vi "Set Config.vi"(8 "error in (no error)":errorcluster, 9 "Variant":variant, 11 "SJ-210 in":refnum<class "SJ-210.lvclass">) -> (0 "error out":errorcluster, 3 "SJ-210 out":refnum<class "SJ-210.lvclass">)   [LabVIEW 2014, in "SJ-210.lvlib" / "SJ-210.lvclass"]
uses:
  SJ-210.lvclass
  SJ-210.lvclass/SJ-210.ctl
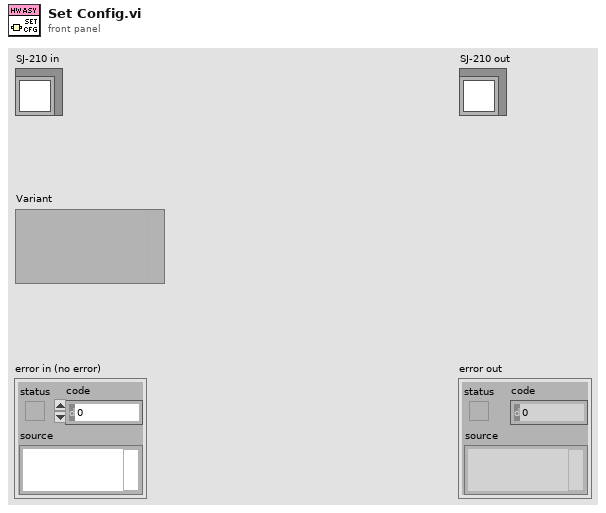
[diagram p1: front panel]
types:
  T1 = cluster{"VISA resource name":refnum<visa-resource-name>}
  T2 = cluster{"Conection Data":cluster{"VISA resource name":refnum<visa-resource-name>}, "ACQ Data":dbl[]}
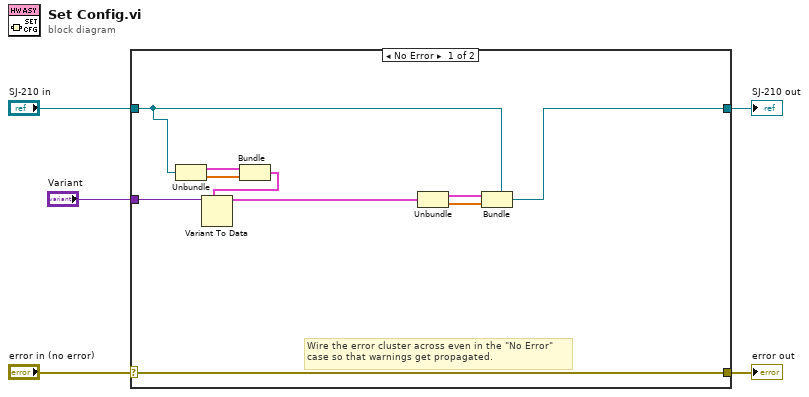
[diagram p0: block diagram]
diagram:
  n1 = case shown="No Error" "error in (no error)" {
    selector: "error in (no error)" -> [w15 w17]
    tunnel: [w15 w17] -> w4
    tunnel: [w11 w16] -> w2
    tunnel: "SJ-210 in" -> [w7 w16]
    tunnel: "Variant" -> [w14 _]
    frame No Error {
      # "Wire the error cluster across even in the \"No Error\"\ncase so that warnings get propagated."
      n2 = Unbundle(w7) -> (w8:T1, w9:dbl[])
      n3 = Bundle("Conection Data"=w8, "ACQ Data"=w9) -> (w6:T2)  [unwired: 1 in]
      n4 = Variant To Data(type=w6, Variant=w14) -> (data=w10:T2)  [unwired: 1 in, 1 out]
      n5 = Unbundle(w10) -> ("Conection Data"=w13:T1, "ACQ Data"=w12:dbl[])
      n6 = Bundle(cluster=w7, w13, w12) -> (w11:refnum<class "SJ-210.lvclass">)
    }
    frame Error {
    }
  }
  "error out" <- w4
  "SJ-210 out" <- w2
